vi "BS1200-Legacy Discovery Parser.vi"(10 "IP Address":string, 11 "Discovery String":string) -> (3 "Devices":T1[](array[typedef]))   [LabVIEW 2021, in "BS120x Driver.lvlib"]
uses:
  BS120x Driver.lvlib
  New BS120x Device/DiscoveredDevice.ctl
  TypeDefs/UnitType.ctl
  TypeDefs/Protocol.ctl
  BS120x.lvclass
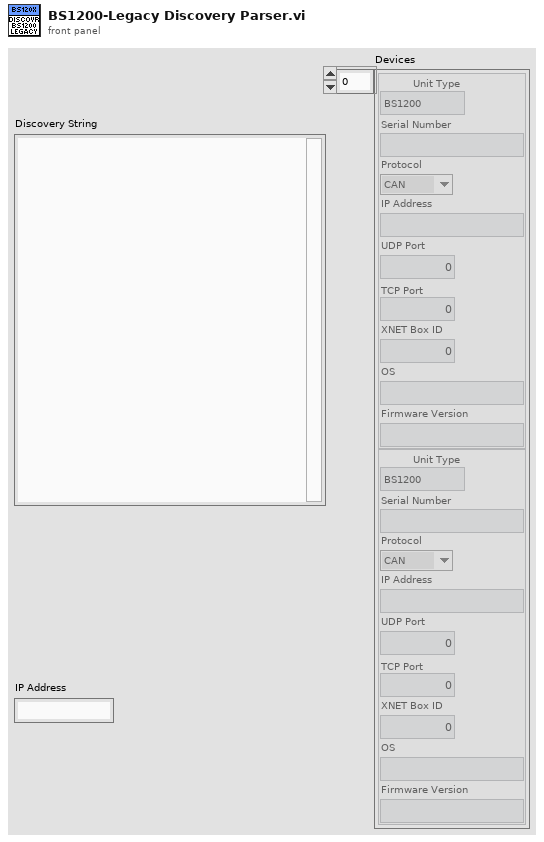
[diagram p1: front panel]
types:
  T1 = typedef "BS120x Driver.lvlib/DiscoveredDevice.ctl" = cluster{"Unit Type":T2, "Serial Number":string, "Protocol":T3, "IP Address":string, "UDP Port":u16, "TCP Port":u16, "XNET Box ID":u8, "OS":string, "Firmware Version":string}
  T2 = typedef "BS120x Driver.lvlib/BS120x.lvclass/UnitType.ctl" = enum16{"BS1200", "BS1201"}
  T3 = typedef "BS120x Driver.lvlib/BS120x.lvclass/Protocol.ctl" = enum16{"CAN", "Ethernet"}
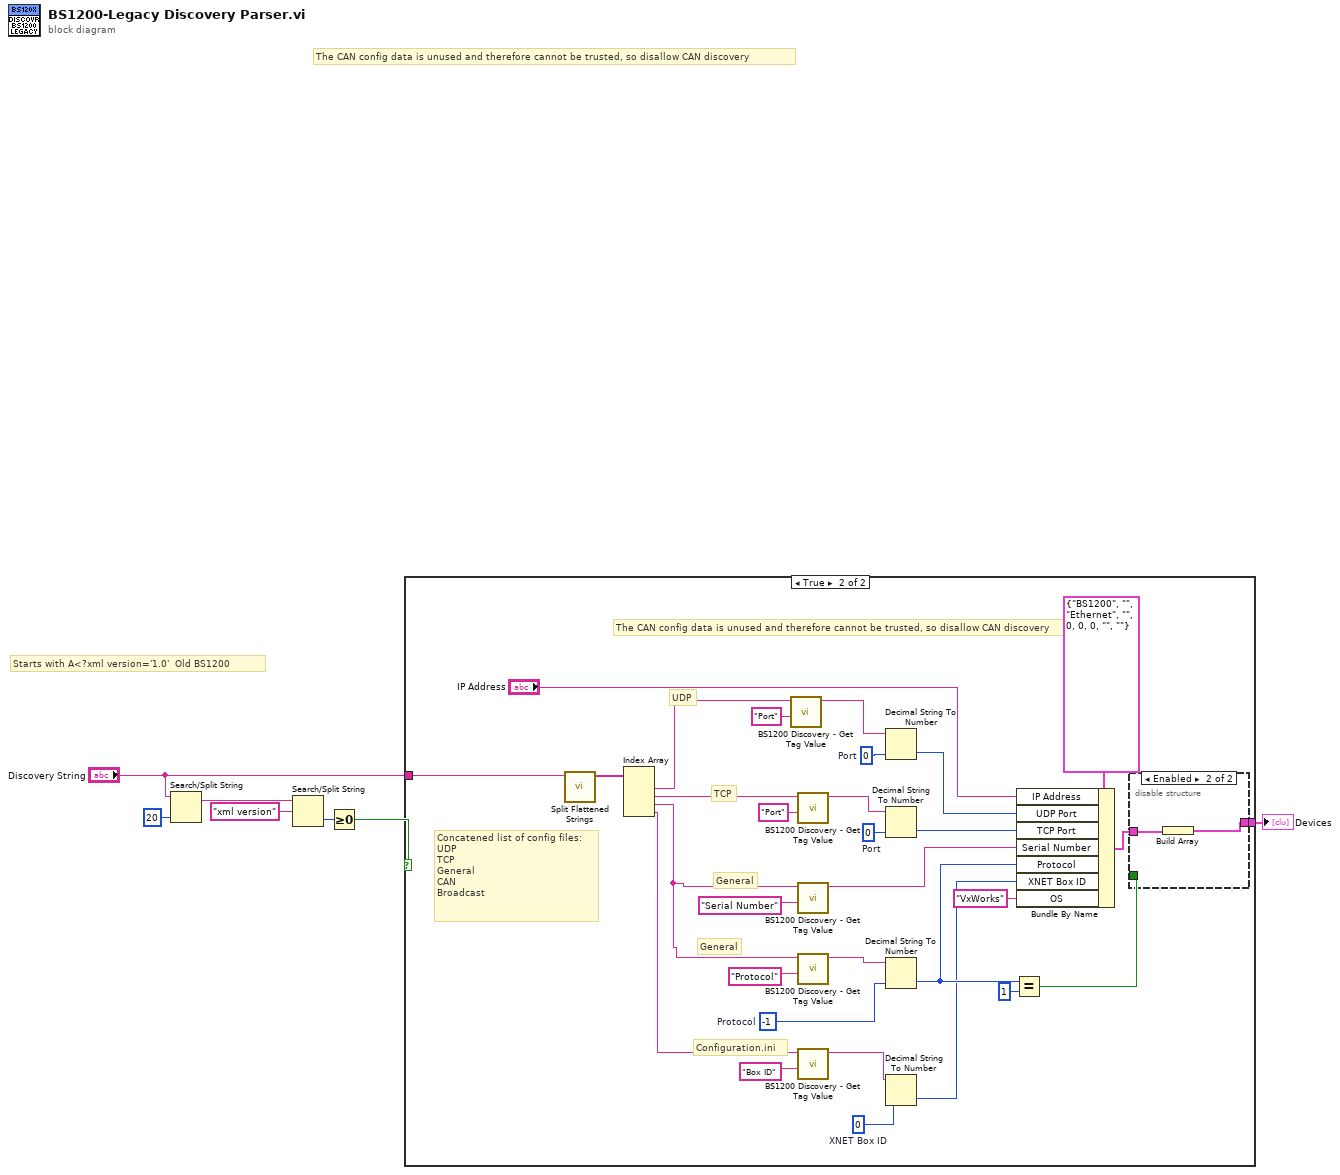
[diagram p0: block diagram]
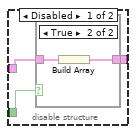
[diagram p3: hidden frame]
diagram:
  # "Starts with A<?xml version='1.0'  Old BS1200"
  # "The CAN config data is unused and therefore cannot be trusted, so disallow CAN discovery"
  n1 = Search/Split String(string="Discovery String", offset (0)=20) -> (substring before match=w4:string)  [unwired: 1 in, 2 out]
  n2 = Search/Split String(string=w4, search string/char (-)="xml version") -> (offset of match=w2:i32)  [unwired: 1 in, 2 out]
  n3 = Greater Or Equal To 0?(x=w2) -> (x >= 0?=w1:bool)
  n4 = case shown="True" w1 {
    tunnel: [_ w27] -> w7
    tunnel: "Discovery String" -> [_ w9]
    frame False {
    }
    frame True {
      w11 = u8 0  # XNET Box ID
      w35 = u16 0  # Port
      w36 = -1  # Protocol
      w38 = u16 0  # Port
      # "Configuration.ini"
      # "General"
      # "General"
      # "TCP"
      # "UDP"
      # "The CAN config data is unused and therefore cannot be trusted, so disallow CAN discovery"
      # "Concatened list of config files:\nUDP\nTCP\nGeneral\nCAN\nBroadcast"
      n5 = call "Split Flattened Strings.vi"("Flattened Strings"=w9) -> ("Strings"=w28:string[])  [unwired: 10 in]
      n6 = Index Array(array=w28) -> (element #1=w26:string, element #2=w22:string, element #3=w20:string, element #4=w15:string)  [unwired: 4 in]
      n7 = call "BS1200 Discovery - Get Tag Value.vi"("Name"="Port", "Input String"=w26) -> ("Value"=w24:string)  [unwired: 9 in]
      n8 = call "BS1200 Discovery - Get Tag Value.vi"("Name"="Port", "Input String"=w22) -> ("Value"=w21:string)  [unwired: 9 in]
      n9 = call "BS1200 Discovery - Get Tag Value.vi"("Name"="Serial Number" ("Initial Filter"), "Input String"=w20) -> ("Value"=w10:string)  [unwired: 9 in]
      n10 = call "BS1200 Discovery - Get Tag Value.vi"("Name"="Protocol" ("Initial Filter"), "Input String"=w20) -> ("Value"=w18:string)  [unwired: 9 in]
      n11 = call "BS1200 Discovery - Get Tag Value.vi"("Name"="Box ID" ("Initial Filter"), "Input String"=w15) -> ("Value"=w13:string)  [unwired: 9 in]
      n12 = Decimal String To Number(string=w24, default (0L)=w38) -> (number=w37:u16)  [unwired: 1 in, 1 out]
      n13 = Decimal String To Number(string=w21, default (0L)=w35) -> (number=w34:u16)  [unwired: 1 in, 1 out]
      n14 = Decimal String To Number(string=w18, default (0L)=w36) -> (number=w14:i32)  [unwired: 1 in, 1 out]
      n15 = Decimal String To Number(string=w13, default (0L)=w11) -> (number=w12:u8)  [unwired: 1 in, 1 out]
      n16 = Equal?(x=w14, y=1) -> (x = y?=w30:bool)
      n17 = Bundle By Name(cluster=T1 {"Unit Type"=enum."BS1200", "Serial Number"="", "Protocol"=enum."Ethernet", "IP Address"="", "UDP Port"=0, "TCP Port"=0, "XNET Box ID"=0, "OS"="", "Firmware Version"=""} ("Device"), "IP Address"="IP Address", "UDP Port"=w37, "TCP Port"=w34, "Serial Number"=w10, "Protocol"=w14, "XNET Box ID"=w12, "OS"="VxWorks" ("Comment")) -> (w31:T1)
      n18 = disable-structure shown="Enabled" {
        disable-tunnel: w31 -> [w41 w45]
        disable-tunnel: w30 -> [w40 _]
        disable-tunnel: [w39 w44] -> w27
        frame Disabled {
          n19 = case shown="True" w40 {
            tunnel: w41 -> [_ w43]
            tunnel: [_ w42] -> w39
            frame False {
            }
            frame True {
              n20 = Build Array(w43) -> (w42:T1[])
            }
          }
        }
        frame Enabled {
          n21 = Build Array(w45) -> (w44:T1[])
        }
      }
    }
  }
  "Devices" <- w7
